vi "Check Free Path.vi"(6 "To Hallway":bool, 7 "Data In":T1, 8 "Hallway Index":i32, 11 "Column":string) -> (0 "Length":i32, 3 "Free Path?":bool)   [LabVIEW 2020]
uses:
  Data.ctl
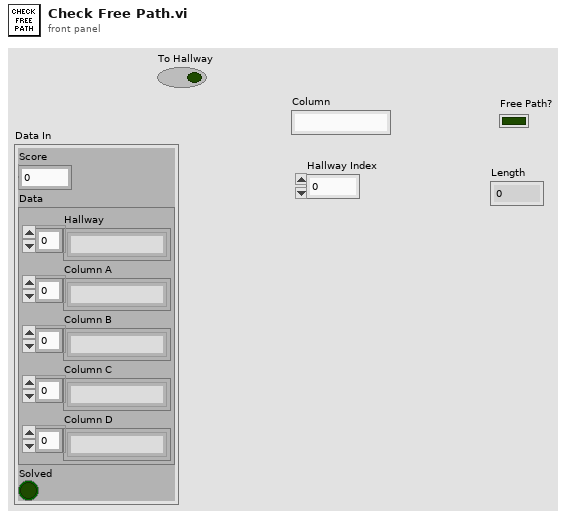
[diagram p1: front panel]
types:
  T1 = typedef "Data.ctl" = cluster{"Score":i64, "Data":cluster{"Hallway":string[], "Column A":string[], "Column B":string[], "Column C":string[], "Column D":string[]}, "Solved":bool}
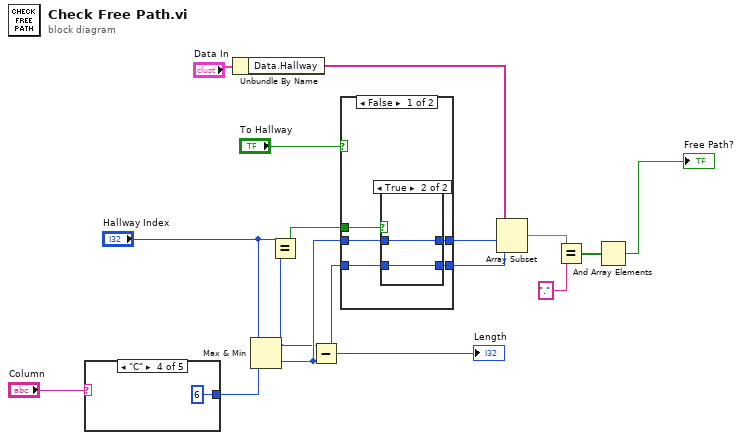
[diagram p0: block diagram]
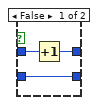
[diagram p2: hidden frame]
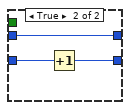
[diagram p3: hidden frame]
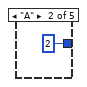
[diagram p5: hidden frame]
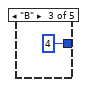
[diagram p6: hidden frame]
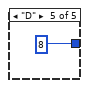
[diagram p7: hidden frame]
diagram:
  n1 = case shown="\"C\"" "Column" {
    tunnel: [_ 2 ("Hallway Index") 4 ("Hallway Index") 6 ("Hallway Index") 8 ("Hallway Index")] -> w15
    frame Default {
    }
    frame "A" {
    }
    frame "B" {
    }
    frame "C" {
    }
    frame "D" {
    }
  }
  n2 = Unbundle By Name("Data In") -> ("Data.Hallway"=w13:string[])
  n3 = Max & Min(x="Hallway Index", y=w15) -> (max(x,y)=w2:i32, min(x,y)=w8:i32)
  n4 = Equal?(x="Hallway Index", y=w2) -> (x = y?=w1:bool)
  n5 = Subtract(x=w2, y=w8) -> (x-y=w5:i32)
  "Length" <- w5
  n6 = case shown="False" "To Hallway" {
    tunnel: w8 -> [w25 w33]
    tunnel: [w24 w33] -> w7
    tunnel: w5 -> [w22 w32]
    tunnel: [w21 w31] -> w4
    tunnel: w1 -> [w23 _]
    frame False {
      n7 = case shown="True" w23 {
        tunnel: w25 -> [w28 w30]
        tunnel: [w27 w30] -> w24
        tunnel: w22 -> [w26 w29]
        tunnel: [w26 w29] -> w21
        frame False {
          n8 = Increment(x=w28) -> (x+1=w27:i32)
        }
        frame True {
        }
      }
    }
    frame True {
      n9 = Increment(x=w32) -> (x+1=w31:i32)
    }
  }
  n10 = Array Subset(array=w13, index=w7, length=w4) -> (w12:string[])
  n11 = Equal?(x=w12, y=".") -> (x = y?=w10:bool[])
  n12 = And Array Elements(Boolean array=w10) -> (logical AND=→"Free Path?":bool)
